vi "Host - Import ESI File.vi"(7 "Select a device profile or file path":path, 8 "error in":errorcluster, 9 "Import to RT target":bool, 10 "Import to host PC":bool, 11 "Target IP Address":string) -> (0 "error out":errorcluster, 3 "result out":string[][](array[string]))   [LabVIEW 2019, in "SEECD System Explorer.lvlib"]
uses:
  SEECD System Explorer.lvlib
  <vilib>/nisyscfg/Close (System).vi
  <vilib>/nisyscfg/nisyscfg.lvlib
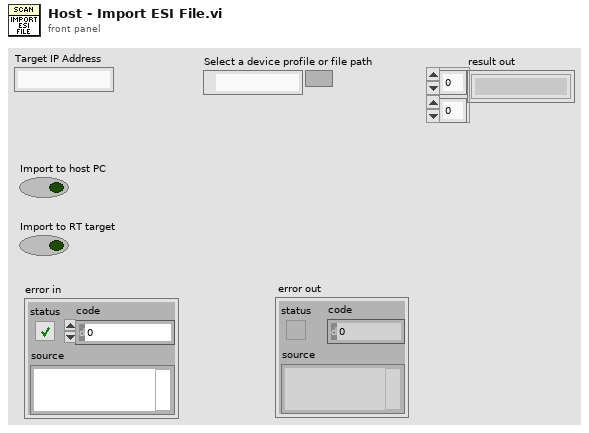
[diagram p1: front panel]
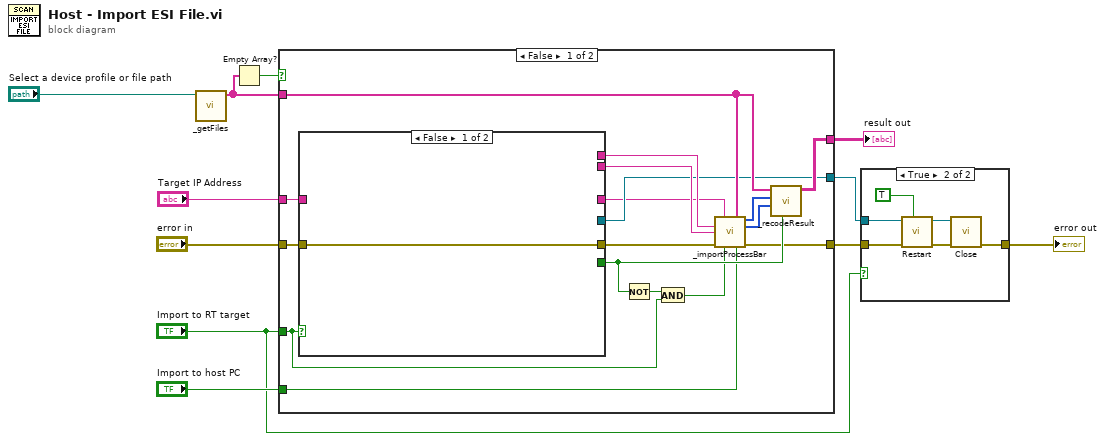
[diagram p0: block diagram]
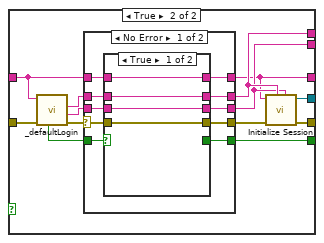
[diagram p3: hidden frame]
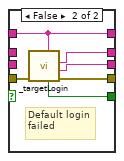
[diagram p4: hidden frame]
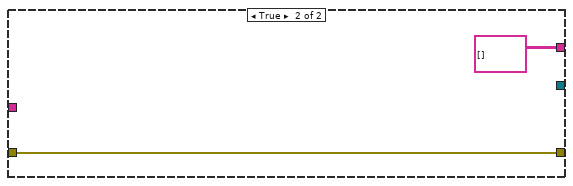
[diagram p6: hidden frame]
diagram:
  n1 = call "_getFiles.vi"("Selected path"="Select a device profile or file path") -> ("Import files"=w6:string[])  [unwired: 6 in]
  n2 = Empty Array?(array=w6) -> (empty?=w7:bool)
  n3 = case shown="False" w7 {
    tunnel: [w28 string[][] [] ("result out")] -> w3
    tunnel: w6 -> [w20 _]
    tunnel: "Target IP Address" -> [w21 _]
    tunnel: "error in" -> [w25 w67]
    tunnel: [w16 _] -> w9
    tunnel: "Import to RT target" -> [w14 _]
    tunnel: "Import to host PC" -> [w13 _]
    tunnel: [w15 w67] -> w4
    frame False {
      n4 = case shown="False" w14 {
        tunnel: w21 -> [_ w37]
        tunnel: [_ w33] -> w24
        tunnel: [_ w32] -> w23
        tunnel: [_ w42] -> w27
        tunnel: [w29 w34] -> w22
        tunnel: w25 -> [w29 w36]
        tunnel: [_ w31] -> w16
        tunnel: [_ w30] -> w12
        frame False {
        }
        frame True {
          n5 = call <resource>:"_defaultLogin.vi"("error in"=w36, "Target IP"=w37) -> ("error out"=w39:errorcluster, "password out"=w40:string, "user name out"=w41:string, "correct login?"=w38:bool)  [unwired: 6 in]
          n6 = case shown="No Error" w39 {
            selector: w39 -> [w46 w66]
            tunnel: [w52 w64] -> w33
            tunnel: [w51 w63] -> w32
            tunnel: [w50 _] -> w42
            tunnel: [w49 w66] -> w35
            tunnel: w41 -> [w48 w64]
            tunnel: w40 -> [w47 w63]
            tunnel: w38 -> [w45 _]
            tunnel: w37 -> [w44 w65]
            tunnel: [w43 w65] -> w30
            frame No Error {
              n7 = case shown="True" w45 {
                tunnel: [w56 w62] -> w52
                tunnel: [w55 w61] -> w51
                tunnel: [w54 w60] -> w49
                tunnel: [_ w59] -> w50
                tunnel: w48 -> [w56 _]
                tunnel: w47 -> [w55 _]
                tunnel: w46 -> [w54 w58]
                tunnel: w44 -> [w53 w57]
                tunnel: [w53 w57] -> w43
                frame True {
                }
                frame False {
                  # "Default login failed"
                  n8 = call <resource>:"_targetLogin.vi"("Target IP"=w57, "error in"=w58) -> ("error out"=w60:errorcluster, "Password out"=w61:string, "Username out"=w62:string, "cancel?"=w59:bool)  [unwired: 6 in]
                }
              }
            }
            frame Error {
            }
          }
          n9 = call <vilib>:"Initialize Session.vi"("Password"=w32, "User Name"=w33, "error in (no error)"=w35, "Target (localhost)"=w30) -> ("error out"=w34:errorcluster, "Session out"=w31:refnum<k21>)  [unwired: 6 in]
        }
      }
      n10 = Not(x=w27) -> (.not. x?=w26:bool)
      n11 = And(x=w26, y=w14) -> (x .and. y?=w17:bool)
      n12 = call "_importProcessBar.vi"("Target IP"=w12, "ProfileSrcPath"=w20, "user name"=w24, "password"=w23, "error in (no error)"=w22, "importTarget?"=w17, "importHost?"=w13) -> ("hostResult"=w19:i32[], "targetResult"=w18:i32[], "error out"=w15:errorcluster)  [unwired: 6 in]
      n13 = call <resource>:"_recodeResult.vi"("cancel?"=w27, "targetResult"=w18, "hostResult"=w19, "Import files"=w20) -> ("result out"=w28:string[][])  [unwired: 7 in]
    }
    frame True {
    }
  }
  "result out" <- w3
  n14 = case shown="True" "Import to RT target" {
    tunnel: w4 -> [w69 w75]
    tunnel: w9 -> [_ w74]
    tunnel: [w69 w70] -> w1
    frame False {
    }
    frame True {
      n15 = call <vilib>:"Restart.vi"("Wait Until Complete (T)"=TRUE, "error in (no error)"=w75, "Session in"=w74) -> ("error out"=w72:errorcluster, "Session out"=w71:refnum<k21>)  [unwired: 6 in, 1 out]
      n16 = call-poly <vilib>:"Close.vi"("error in (no error)"=w72, "Session in"=w71) -> ("error out"=w70:errorcluster)  [unwired: 9 in]
    }
  }
  "error out" <- w1
